vi "niFPGA Trigger_m.vi"   [LabVIEW 2017]
doc: "Detects changes of the input signal during a control or simulation process. The data type you wire to <B>trigger signal</B> determines the <B>triggered</B> data type."
uses:
  <vilib>/rvi/Analysis/common/FxpNativeNode/niFpgaFxpNative.xnode
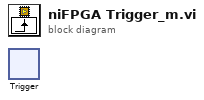
[diagram p0: block diagram]
diagram:
  n1 = xnode "Trigger"() -> ()  [unwired: 3 in, 1 out]
